vi "Move To Raw.vi"(6 "Destination Angle":dbl=nan, 7 "Wait?":bool=TRUE, 8 "error in":errorcluster, 9 "Speed":dbl=5.0, 10 "Destination":refnum<class "Vec3d.lvclass">, 11 "Gantry in":refnum<class "Gantry.lvclass">) -> (0 "error out":errorcluster, 3 "Gantry out":refnum<class "Gantry.lvclass">)   [LabVIEW 2026, in "Gantry.lvclass"]
uses:
  Gantry.lvclass
  Vec3d Class/Vec3d.lvclass
  Gantry.lvclass/Gantry.ctl
  <instrlib>/Aerotech Automation1/Commands/Motion/typedefs/MoveLinear parameters.ctl
  <instrlib>/Aerotech Automation1/Aerotech Automation1.lvlib
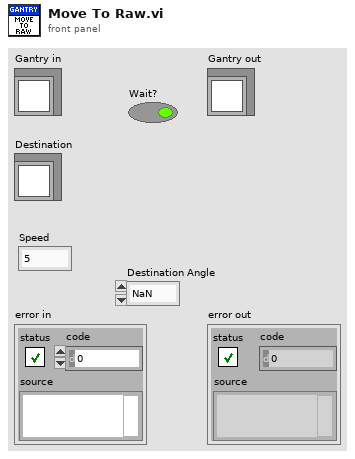
[diagram p1: front panel]
types:
  T1 = typedef "Aerotech Automation1.lvlib/MoveLinear parameters.ctl" = cluster{"coordinatedSpeed":dbl, "distances":dbl[], "axes":string[]}
  T2 = typedef "Virtual Modes.ctl" = enum16{"Nonvirtual", "Virtual"}
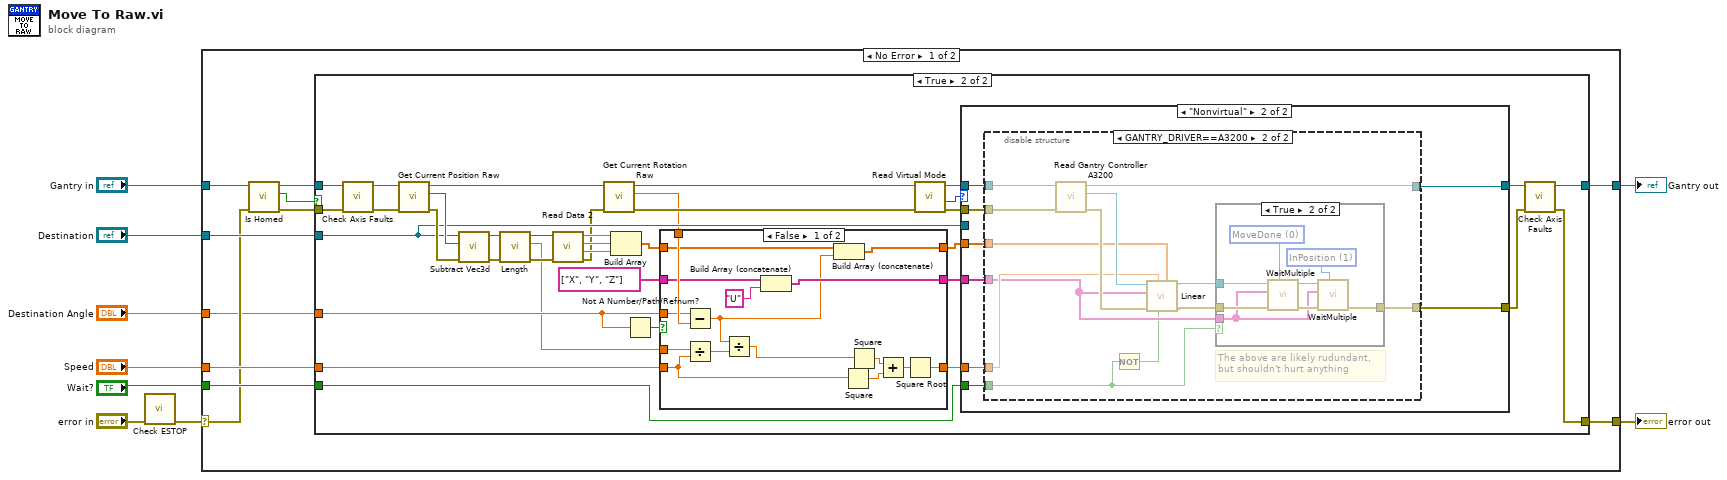
[diagram p0: block diagram]
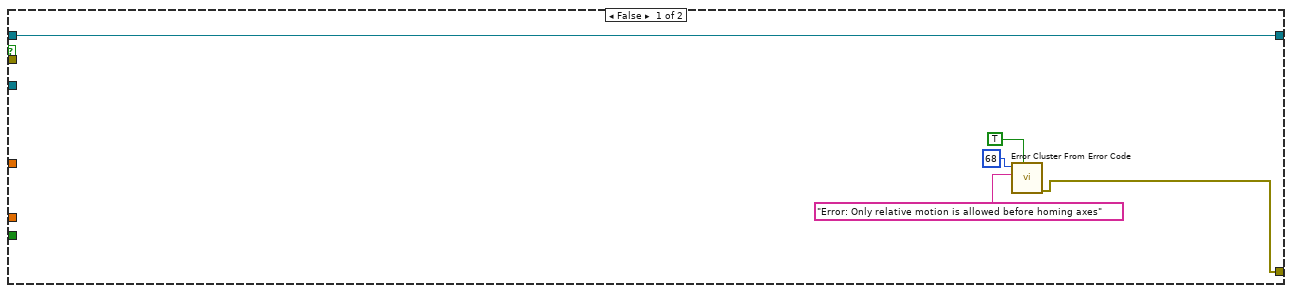
[diagram p2: hidden frame]
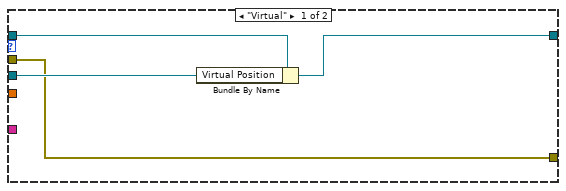
[diagram p4: hidden frame]
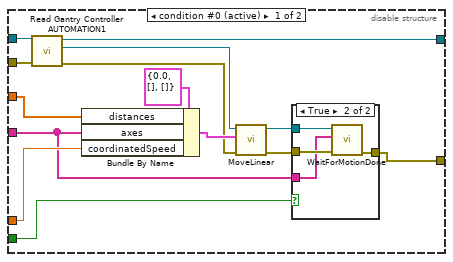
[diagram p5: hidden frame]
diagram:
  n1 = call "Check ESTOP.vi"("error in"="error in") -> ("error out"=w3:errorcluster)  [unwired: 10 in]
  n2 = case shown="No Error" w3 {
    selector: w3 -> [w12 w135]
    tunnel: [w16 w135] -> w9
    tunnel: [w17 w134] -> w8
    tunnel: "Gantry in" -> [w15 w134]
    tunnel: "Destination" -> [w19 _]
    tunnel: "Wait?" -> [w20 _]
    tunnel: "Speed" -> [w18 _]
    tunnel: "Destination Angle" -> [w10 _]
    frame No Error {
      n3 = call "Is Homed.vi"("error in (no error)"=w12, "Gantry in"=w15) -> ("error out"=w11:errorcluster, "homed?"=w13:bool, "Gantry out"=w14:refnum<class "Gantry.lvclass">)  [unwired: 7 in]
      n4 = case shown="True" w13 {
        tunnel: w20 -> [_ w44]
        tunnel: w19 -> [_ w45]
        tunnel: w14 -> [w21 w49]
        tunnel: w18 -> [_ w39]
        tunnel: w11 -> [_ w47]
        tunnel: [w21 w52] -> w17
        tunnel: [w22 w50] -> w16
        tunnel: w10 -> [_ w42]
        frame False {
          n5 = call <vilib>:"Error Cluster From Error Code.vi"("show call chain? (False)"=TRUE, "error message (\"\")"="Error: Only relative motion is allowed before homing axes", "error code (0)"=68) -> ("error out"=w22:errorcluster)  [unwired: 6 in]
        }
        frame True {
          n6 = call "Check Axis Faults.vi"("error in (no error)"=w47, "Gantry in"=w49) -> ("error out"=w46:errorcluster, "Gantry out"=w48:refnum<class "Gantry.lvclass">)  [unwired: 8 in]
          n7 = call-dynamic "Get Current Position Raw.vi"("error in"=w46, "Gantry in"=w48) -> ("error out"=w57:errorcluster, "Vec3d Class out"=w58:refnum<class "Vec3d.lvclass">, "Gantry out"=w35:refnum<class "Gantry.lvclass">)  [unwired: 7 in]
          n8 = call "Subtract Vec3d.vi"("error in (no error)"=w57, "Vec3d in 2"=w58, "Vec3d in 1"=w45) -> ("error out"=w29:errorcluster, "Vec3d Class out"=w30:refnum<class "Vec3d.lvclass">)  [unwired: 7 in]
          n9 = call-dynamic "Length.vi"("error in"=w29, "Vec3d in"=w30) -> ("error out"=w28:errorcluster, "Length"=w26:dbl, "Vec3d out"=w27:refnum<class "Vec3d.lvclass">)  [unwired: 7 in]
          n10 = call-dynamic "Read Data 2.vi"("error in"=w28, "Vec3d in"=w27) -> ("error out"=w34:errorcluster, "Z"=w54:dbl, "Y"=w55:dbl, "X"=w56:dbl)  [unwired: 6 in]
          n11 = call-dynamic "Get Current Rotation Raw.vi"("error in"=w34, "Gantry in"=w35) -> ("error out"=w32:errorcluster, "Current Rotation"=w31:dbl, "Gantry out"=w33:refnum<class "Gantry.lvclass">)  [unwired: 7 in]
          n12 = Build Array(w56, w55, w54) -> (w41:dbl[])
          n13 = Not A Number/Path/Refnum?(number/path/refnum=w42) -> (NaN/Path/Refnum?=w43:bool)
          n14 = case shown="False" w43 {
            tunnel: w42 -> [w76 _]
            tunnel: w41 -> [w65 w79]
            tunnel: string[] ["X", "Y", "Z"] -> [w67 w78]
            tunnel: w39 -> [w70 w80]
            tunnel: [w72 w80] -> w38
            tunnel: [w64 w79] -> w37
            tunnel: [w63 w78] -> w36
            tunnel: w31 -> [w77 _]
            tunnel: w26 -> [w71 _]
            frame False {
              n15 = Subtract(x=w76, y=w77) -> (x-y=w62:dbl)
              n16 = Divide(x=w71, y=w70) -> (x/y=w69:dbl)
              n17 = Divide(x=w62, y=w69) -> (x/y=w68:dbl)
              n18 = Build Array (concatenate)(w67, "U") -> (w63:string[])
              n19 = Build Array (concatenate)(w65, w62) -> (w64:dbl[])
              n20 = Square(x=w70) -> (x^2=w75:dbl)
              n21 = Square(x=w68) -> (x^2=w74:dbl)
              n22 = Add(x=w74, y=w75) -> (x+y=w73:dbl)
              n23 = Square Root(x=w73) -> (sqrt(x)=w72:dbl)
            }
            frame True {
            }
          }
          n24 = call-dynamic "Read Virtual Mode.vi"("error in (no error)"=w32, "Gantry in"=w33) -> ("error out"=w59:errorcluster, "Virtual Mode"=w60:T2, "Gantry out"=w61:refnum<class "Gantry.lvclass">)  [unwired: 6 in, 1 out]
          n25 = case shown="\"Nonvirtual\"" w60 {
            tunnel: w44 -> [_ w90]
            tunnel: w61 -> [w84 w92]
            tunnel: [w81 w89] -> w53
            tunnel: [w82 w88] -> w51
            tunnel: w59 -> [w82 w91]
            tunnel: w38 -> [_ w85]
            tunnel: w37 -> [_ w87]
            tunnel: w36 -> [_ w86]
            tunnel: w45 -> [w83 _]
            frame "Virtual" {
              n26 = Bundle By Name(cluster=w84, "Virtual Position"=w83) -> (w81:refnum<class "Gantry.lvclass">)
            }
            frame "Nonvirtual" {
              n27 = disable-structure shown="GANTRY_DRIVER==A3200" {
                disable-tunnel: w92 -> [w106 w124]
                disable-tunnel: w91 -> [w105 w123]
                disable-tunnel: w90 -> [w104 w113]
                disable-tunnel: [w98 w116] -> w89
                disable-tunnel: [w99 w115] -> w88
                disable-tunnel: w87 -> [w102 w117]
                disable-tunnel: w86 -> [w97 w114]
                disable-tunnel: w85 -> [w101 w118]
                frame condition #0 (active) {
                  n28 = call "Read Gantry Controller AUTOMATION1.vi"("error in (no error)"=w105, "Gantry in"=w106) -> ("error out"=w95:errorcluster, "Controller AUTOMATION1"=w96:refnum<k24>, "Gantry out"=w98:refnum<class "Gantry.lvclass">)  [unwired: 7 in]
                  n29 = Bundle By Name(cluster=T1 {"coordinatedSpeed"=0.0, "distances"=[], "axes"=[]} ("MoveLinear parameters"), "distances"=w102, "axes"=w97, "coordinatedSpeed"=w101) -> (w100:T1)
                  n30 = call <instrlib>:"MoveLinear.vi"("error in (no error)"=w95, "MoveLinear parameters"=w100, "Controller Refnum"=w96) -> ("error out"=w93:errorcluster, "Controller Refnum out"=w94:refnum<k24>)  [unwired: 7 in]
                  n31 = case shown="True" w104 {
                    tunnel: w94 -> [_ w111]
                    tunnel: w93 -> [w107 w110]
                    tunnel: [w107 w109] -> w99
                    tunnel: w97 -> [_ w108]
                    frame False {
                    }
                    frame True {
                      n32 = call <instrlib>:"WaitForMotionDone.vi"("error in (no error)"=w110, "axes"=w108, "Controller Refnum"=w111) -> ("error out"=w109:errorcluster)  [unwired: 7 in, 1 out]
                    }
                  }
                }
                frame condition #1 {
                  # "The above are likely rudundant,\nbut shouldn't hurt anything"
                  n33 = call "Read Gantry Controller A3200.vi"("error in (no error)"=w123, "Gantry in"=w124) -> ("error out"=w120:errorcluster, "A3200 controller out"=w119:refnum<k24>, "Gantry out"=w116:refnum<class "Gantry.lvclass">)  [unwired: 7 in]
                  n34 = Not(x=w113) -> (.not. x?=w112:bool)
                  n35 = call "Linear.vi"("distances"=w117, "return immediately"=w112, "speed"=w118, "error in (no error)"=w120, "axis names"=w114, "controller in"=w119) -> ("error out"=w121:errorcluster, "controller out"=w122:refnum<k24>)  [unwired: 4 in]
                  n36 = case shown="True" w113 {
                    tunnel: w122 -> [_ w133]
                    tunnel: w121 -> [w125 w132]
                    tunnel: [w125 w130] -> w115
                    tunnel: w114 -> [_ w126]
                    frame False {
                    }
                    frame True {
                      w127 = 1 items=["MoveDone", "InPosition"] ("wait option?")
                      w128 = 0 items=["MoveDone", "InPosition"] ("wait option?")
                      n37 = call "WaitMultiple.vi"("wait option?"=w128, "error in (no error)"=w132, "axis names"=w126, "controller in"=w133) -> ("error out"=w131:errorcluster, "controller out"=w129:refnum<k24>)  [unwired: 5 in, 1 out]
                      n38 = call "WaitMultiple.vi"("wait option?"=w127, "error in (no error)"=w131, "axis names"=w126, "controller in"=w129) -> ("error out"=w130:errorcluster)  [unwired: 5 in, 2 out]
                    }
                  }
                }
              }
            }
          }
          n39 = call "Check Axis Faults.vi"("error in (no error)"=w51, "Gantry in"=w53) -> ("error out"=w50:errorcluster, "Gantry out"=w52:refnum<class "Gantry.lvclass">)  [unwired: 8 in]
        }
      }
    }
    frame Error {
    }
  }
  "error out" <- w9
  "Gantry out" <- w8
